vi "get connection string.vi"(11 "connection client in":refnum<class "connection client.lvclass">) -> (3 "connection string":string)   [LabVIEW 2015, in "connection client.lvclass"]
uses:
  connection client.lvclass
  connection client.lvclass/connection client.ctl
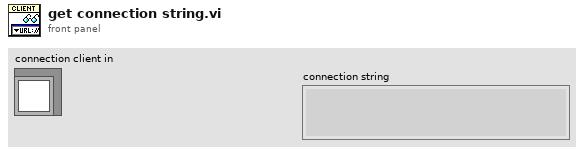
[diagram p1: front panel]
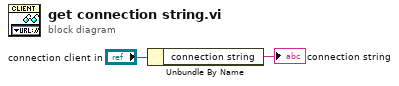
[diagram p0: block diagram]
diagram:
  n1 = Unbundle By Name("connection client in") -> ("connection string"=→"connection string":string)
